vi "Bot.vi"(7 "BotData":T3, 11 "GameState":T1) -> (0 "error out":errorcluster, 3 "Move":T4)   [LabVIEW 2015, in "TronVIEWBotAPI.lvlib"]
uses:
  TronVIEWBotAPI.lvlib
  MovementDirection.ctl
  BotData.ctl
  GameState.ctl
  TronviewGame/Board/Position.ctl
  TronviewGame/Board/Board.lvclass
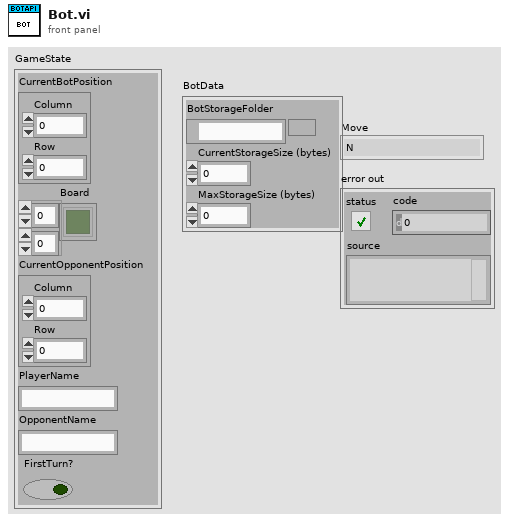
[diagram p1: front panel]
types:
  T1 = typedef "TronVIEWBotAPI.lvlib/GameState.ctl" = cluster{"CurrentBotPosition":T2, "Board":bool[][], "CurrentOpponentPosition":T2, "PlayerName":string, "OpponentName":string, "FirstTurn?":bool}
  T2 = typedef "TronviewGame.lvlib/Board.lvclass/Position.ctl" = cluster{"Column":i32, "Row":i32}
  T3 = typedef "TronVIEWBotAPI.lvlib/BotData.ctl" = cluster{"BotStorageFolder":path, "CurrentStorageSize (bytes)":i64, "MaxStorageSize (bytes)":i64}
  T4 = typedef "TronVIEWBotAPI.lvlib/MovementDirection.ctl" = enum16{"N", "S", "W", "E"}
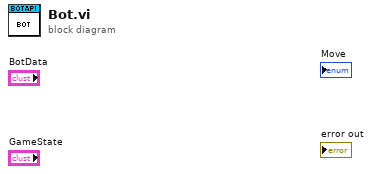
[diagram p0: block diagram]
diagram:
